vi "TagWrite.vi"(7 "LabVIEW Web Service Request":refnum<class "Web Request.lvclass">, 9 "value":T3="0", 10 "tagName":T1, 11 "type":T2) -> ()   [LabVIEW 2013]
uses:
  <vilib>/wsapi/Web Request.lvclass
  <vilib>/NI/TagWebClient/API/String Controls/value.ctl
  <vilib>/NI/TagWebClient/API/String Controls/type.ctl
  <vilib>/NI/TagWebClient/API/String Controls/tagName.ctl
  <vilib>/NI/Tag Bus/tag/Data Type.ctl
  <vilib>/NI/Tag Bus/table/data polymorphs/write one/write Double.vi
  <vilib>/NI/Tag Bus/table/data polymorphs/write one/write Single.vi
  <vilib>/NI/Tag Bus/table/data polymorphs/write one/write I64.vi
  <vilib>/NI/Tag Bus/table/data polymorphs/write one/write I32.vi
  <vilib>/NI/Tag Bus/table/data polymorphs/write one/write I16.vi
  <vilib>/NI/Tag Bus/table/data polymorphs/write one/write I8.vi
  <vilib>/NI/Tag Bus/table/data polymorphs/write one/write U64.vi
  <vilib>/NI/Tag Bus/table/data polymorphs/write one/write U32.vi
  <vilib>/NI/Tag Bus/table/data polymorphs/write one/write U16.vi
  <vilib>/NI/Tag Bus/table/data polymorphs/write one/write U8.vi
  <vilib>/NI/Tag Bus/table/data polymorphs/write one/write String.vi
  <vilib>/NI/Tag Bus/table/data polymorphs/write one/write Boolean.vi
  <vilib>/NI/Tag Bus/table/data table.lvlib
  <vilib>/NI/Tag Bus/tag/tag descriptor.lvclass
  <vilib>/NI/Tag Bus/dictionary/data dictionary.lvclass
  <vilib>/NI/TagWebClient/API/tagweb client API.lvlib
panel:
  # "Use the Web Service Request input terminal to call the VIs on the Web Services palette. Do not remove it from the connector pane unless you don't need access to the palette."
  # "Each additional control wired to the connector pane will be available as an input in the URL. To include an indicator in terminal-mode output (the default setting), it must also be wired to the connector pane."
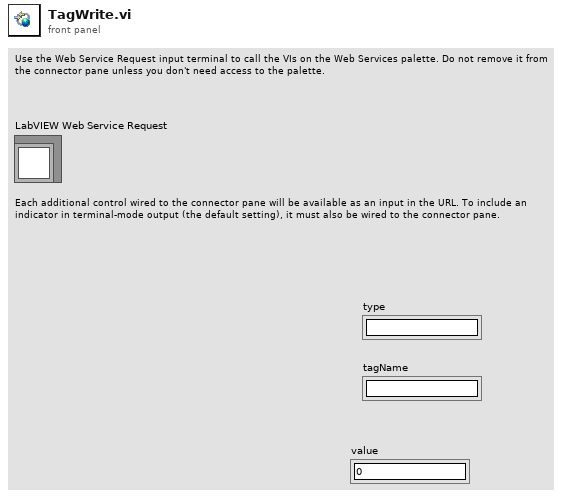
[diagram p1: front panel]
types:
  T1 = typedef "tagweb client API.lvlib/tagName.ctl" = string
  T2 = typedef "tagweb client API.lvlib/type.ctl" = string
  T3 = typedef "tagweb client API.lvlib/value.ctl" = string
  T4 = typedef "tag bus.lvlib/tag descriptor.lvclass/Data Type.ctl" = enum16{"Double", "Single", "I64", "I32", "I16", "I8", "U64", "U32", "U16", "U8", "Boolean", "String", "Array of Double", "Array of Single", "Array of I64", "Array of I32", "Array of I16", "Array of I8", "Array of U64", "Array of U32", "Array of U16", "Array of U8", "Array of Boolean", "Array of String"}
  T5 = typedef "tag bus.lvlib/data table.lvlib/data table.ctl" = cluster{"Double":dbl[], "Single":sgl[], "I64":i64[], "I32":i32[], "I16":i16[], "I8":i8[], "U64":u64[], "U32":u32[], "U16":u16[], "U8":u8[], "Boolean":bool[], "String":string[], "Array of Double":cluster{"DBL Array":dbl[]}[], "Array of Single":cluster{"SGL Array":sgl[]}[], "Array of I64":cluster{"I64 Array":i64[]}[], "Array of I32":cluster{"I32 Array":i32[]}[], "Array of I16":cluster{"I16 Array":i16[]}[], "Array of I8":cluster{"I8 Array":i8[]}[], "Array of U64":cluster{"U64 Array":u64[]}[], "Array of U32":cluster{"U32 Array":u32[]}[], "Array of U16":cluster{"U16 Array":u16[]}[], "Array of U8":cluster{"U8 Array":u8[]}[], "Array of Boolean":cluster{"Boolean Array":bool[]}[], "Array of String":cluster{"String Array":string[]}[]}
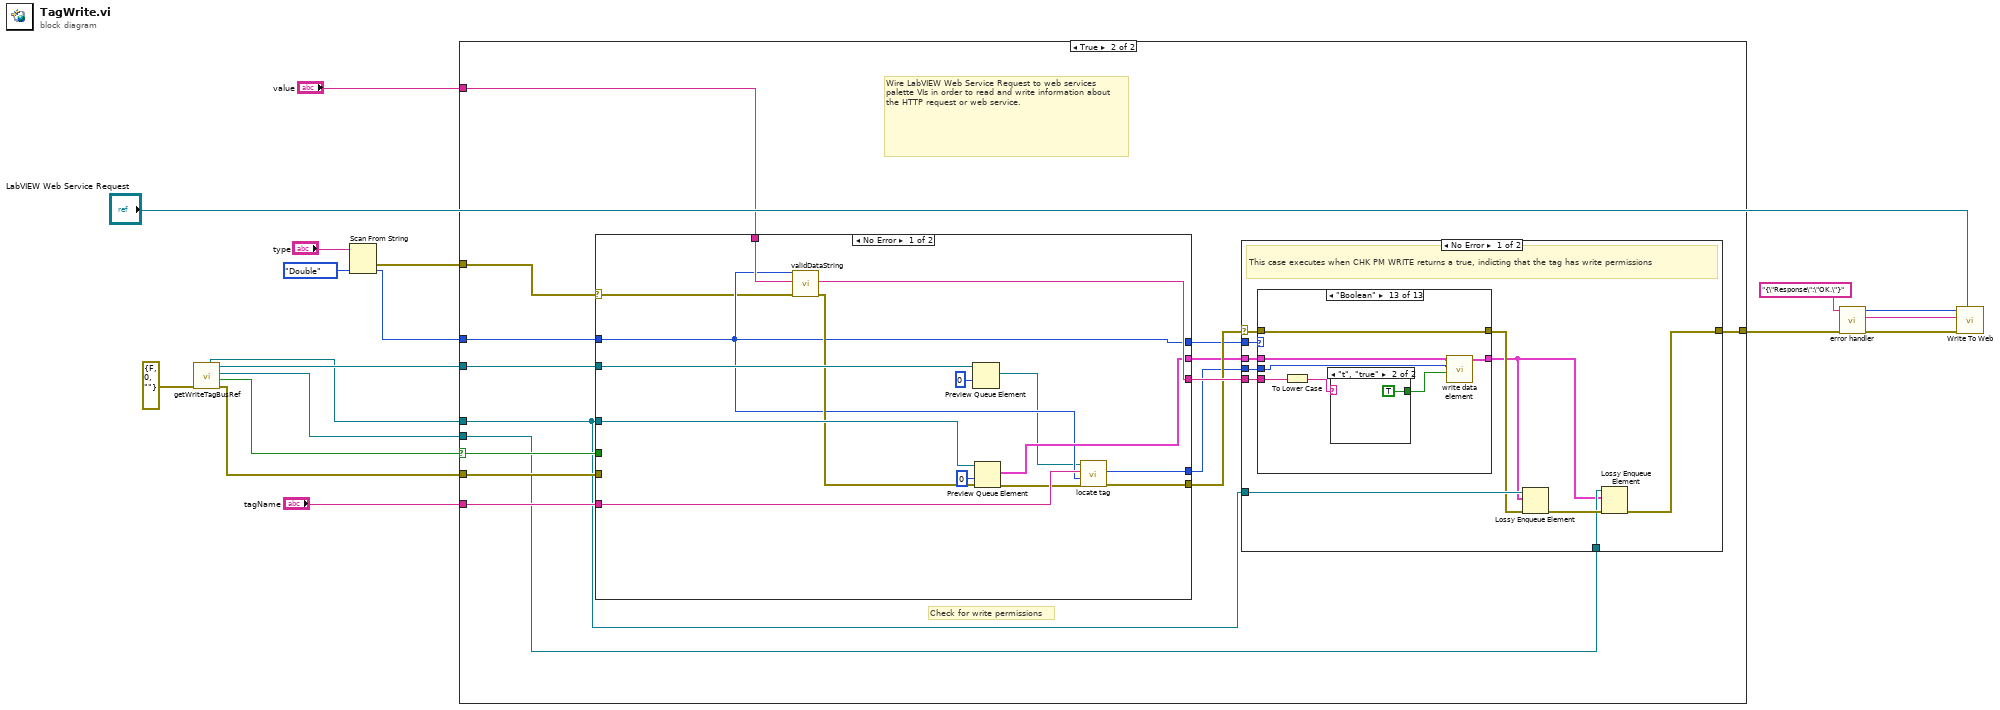
[diagram p0: block diagram]
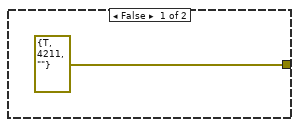
[diagram p2: hidden frame]
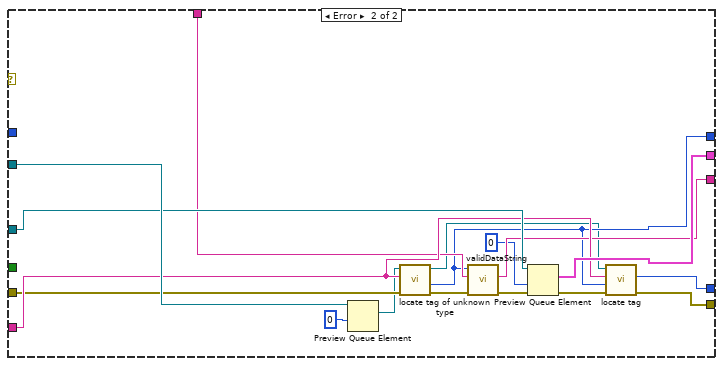
[diagram p3: hidden frame]
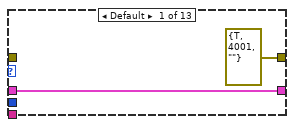
[diagram p4: hidden frame]
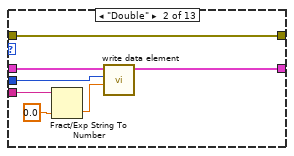
[diagram p5: hidden frame]
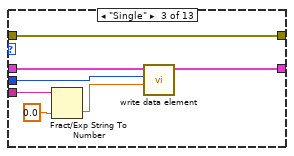
[diagram p6: hidden frame]
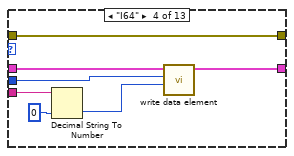
[diagram p7: hidden frame]
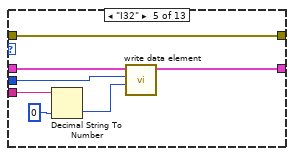
[diagram p8: hidden frame]
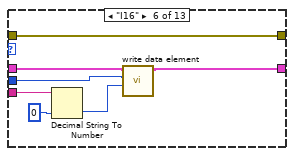
[diagram p9: hidden frame]
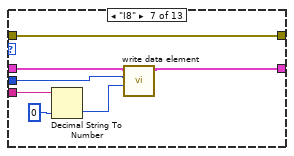
[diagram p10: hidden frame]
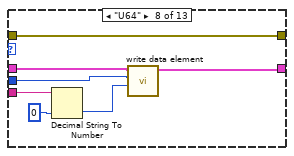
[diagram p11: hidden frame]
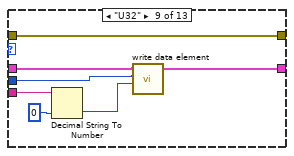
[diagram p12: hidden frame]
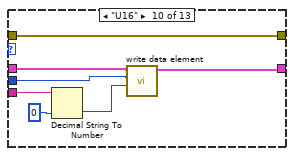
[diagram p13: hidden frame]
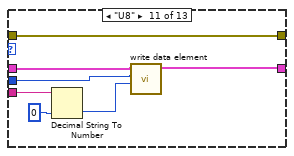
[diagram p14: hidden frame]
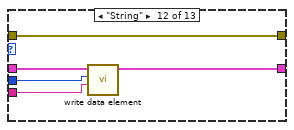
[diagram p15: hidden frame]
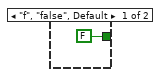
[diagram p16: hidden frame]
diagram:
  n1 = call "getWriteTagBusRef.vi"("error in"=errorcluster {"status"=FALSE, "code"=0, "source"=""} ("error in (no error)")) -> ("error out"=w14:errorcluster, "valid references"=w1:bool, "write tx data table"=w6:refnum<queue>, "write data dictionary"=w15:refnum<queue>, "actual write data table"=w7:refnum<queue>)  [unwired: 6 in]
  n2 = Scan From String(input string="type", default 1=Data_Type."Double" ("data type")) -> (error out=w9:errorcluster, output 1=w8:T4)  [unwired: 3 in, 2 out]
  n3 = case shown="True" w1 {
    selector: w1 -> [_ w22]
    tunnel: [errorcluster {"status"=TRUE, "code"=4211, "source"=""} ("error IO") w34] -> w18
    tunnel: w15 -> [_ w33]
    tunnel: w14 -> [_ w27]
    tunnel: "value" -> [_ w26]
    tunnel: "tagName" -> [_ w25]
    tunnel: w9 -> [_ w24]
    tunnel: w8 -> [_ w23]
    tunnel: w7 -> [_ w20]
    tunnel: w6 -> [_ w21]
    frame False {
    }
    frame True {
      # "Check for write permissions"
      # "Wire LabVIEW Web Service Request to web services palette VIs in order to read and write information about the HTTP request or web service."
      n4 = case shown="No Error" w24 {
        selector: w24 -> [w35 _]
        tunnel: w26 -> [w49 w60]
        tunnel: w33 -> [w48 w66]
        tunnel: w20 -> [w47 w65]
        tunnel: [w46 w59] -> w32
        tunnel: w22 -> [_ _]
        tunnel: w25 -> [w44 w61]
        tunnel: [w43 w64] -> w31
        tunnel: [w40 w58] -> w30
        tunnel: [w42 w63] -> w29
        tunnel: [w41 w62] -> w28
        tunnel: w27 -> [_ w57]
        tunnel: w23 -> [w40 _]
        frame No Error {
          n5 = call "validDataString.vi"("error in (no error)"=w35, "value in"=w49, "data type"=w40) -> ("error out"=w45:errorcluster, "value out"=w46:string)  [unwired: 6 in, 1 out]
          n6 = Preview Queue Element(queue=w48, timeout in ms (-1)=0) -> (element=w36:refnum<class "data dictionary.lvclass">)  [unwired: 1 in, 3 out]
          n7 = Preview Queue Element(queue=w47, timeout in ms (-1)=0, error in (no error)=w45) -> (element=w41:T5, error out=w38:errorcluster)  [unwired: 2 out]
          n8 = call <vilib>:"locate tag.vi"("error in"=w38, "data type"=w40, "name"=w44, "data dictionary in"=w36) -> ("error out"=w43:errorcluster, "index"=w42:i32)  [unwired: 5 in, 1 out]
        }
        frame Error {
          n9 = Preview Queue Element(queue=w66, timeout in ms (-1)=0) -> (element=w50:refnum<class "data dictionary.lvclass">)  [unwired: 1 in, 3 out]
          n10 = call <vilib>:"locate tag of unknown type.vi"("error in"=w57, "name"=w61, "data dictionary in"=w50) -> ("error out"=w52:errorcluster, "data type"=w58:T4, "data dictionary out"=w51:refnum<class "data dictionary.lvclass">)  [unwired: 5 in, 1 out]
          n11 = call "validDataString.vi"("error in (no error)"=w52, "value in"=w60, "data type"=w58) -> ("error out"=w53:errorcluster, "value out"=w59:string)  [unwired: 6 in, 1 out]
          n12 = Preview Queue Element(queue=w65, timeout in ms (-1)=0, error in (no error)=w53) -> (element=w62:T5, error out=w55:errorcluster)  [unwired: 2 out]
          n13 = call <vilib>:"locate tag.vi"("error in"=w55, "data type"=w58, "name"=w61, "data dictionary in"=w51) -> ("error out"=w64:errorcluster, "index"=w63:i32)  [unwired: 5 in, 1 out]
        }
      }
      n14 = case shown="No Error" w31 {
        selector: w31 -> [w73 w164]
        tunnel: w32 -> [w77 _]
        tunnel: w29 -> [w76 _]
        tunnel: [w69 w164] -> w34
        tunnel: w30 -> [w75 _]
        tunnel: w28 -> [w74 _]
        tunnel: w20 -> [w72 _]
        tunnel: w21 -> [w68 _]
        frame No Error {
          # "This case executes when CHK PM WRITE returns a true, indicting that the tag has write permissions"
          n15 = case shown="\"Boolean\"" w75 {
            tunnel: w76 -> [_ w83 w88 w95 w102 w109 w116 w124 w131 w137 w144 w152 w156]
            tunnel: [errorcluster {"status"=TRUE, "code"=4001, "source"=""} ("error out") w81 w91 w98 w105 w112 w119 w126 w133 w140 w147 w154 w159] -> w71
            tunnel: w77 -> [_ w86 w93 w100 w107 w114 w121 w128 w135 w142 w149 w151 w161]
            tunnel: w74 -> [w78 w84 w90 w97 w103 w110 w117 w125 w132 w139 w145 w153 w158]
            tunnel: w73 -> [_ w81 w91 w98 w105 w112 w119 w126 w133 w140 w147 w154 w159]
            tunnel: [w78 w80 w89 w96 w104 w111 w118 w122 w129 w138 w146 w150 w157] -> w67
            frame Default {
            }
            frame "Double" {
              n16 = Fract/Exp String To Number(string=w86, default (0 dbl)=0.0 ("Value")) -> (number=w82:dbl)  [unwired: 2 in, 1 out]
              n17 = call-poly <vilib>:"write data element.vi"("value"=w82, "index"=w83, "data table in"=w84) -> ("data table out"=w80:T5)  [unwired: 8 in]
            }
            frame "Single" {
              n18 = Fract/Exp String To Number(string=w93, default (0 dbl)=sgl 0.0 ("Value")) -> (number=w87:sgl)  [unwired: 2 in, 1 out]
              n19 = call-poly <vilib>:"write data element.vi"("value"=w87, "index"=w88, "data table in"=w90) -> ("data table out"=w89:T5)  [unwired: 8 in]
            }
            frame "I64" {
              n20 = Decimal String To Number(string=w100, default (0L)=i64 0 ("Value")) -> (number=w94:i64)  [unwired: 1 in, 1 out]
              n21 = call-poly <vilib>:"write data element.vi"("value"=w94, "index"=w95, "data table in"=w97) -> ("data table out"=w96:T5)  [unwired: 8 in]
            }
            frame "I32" {
              n22 = Decimal String To Number(string=w107, default (0L)=0 ("Value")) -> (number=w101:i32)  [unwired: 1 in, 1 out]
              n23 = call-poly <vilib>:"write data element.vi"("value"=w101, "index"=w102, "data table in"=w103) -> ("data table out"=w104:T5)  [unwired: 8 in]
            }
            frame "I16" {
              n24 = Decimal String To Number(string=w114, default (0L)=i16 0 ("Value")) -> (number=w108:i16)  [unwired: 1 in, 1 out]
              n25 = call-poly <vilib>:"write data element.vi"("value"=w108, "index"=w109, "data table in"=w110) -> ("data table out"=w111:T5)  [unwired: 8 in]
            }
            frame "I8" {
              n26 = Decimal String To Number(string=w121, default (0L)=i8 0 ("Value")) -> (number=w115:i8)  [unwired: 1 in, 1 out]
              n27 = call-poly <vilib>:"write data element.vi"("value"=w115, "index"=w116, "data table in"=w117) -> ("data table out"=w118:T5)  [unwired: 8 in]
            }
            frame "U64" {
              n28 = Decimal String To Number(string=w128, default (0L)=u64 0 ("Value")) -> (number=w123:u64)  [unwired: 1 in, 1 out]
              n29 = call-poly <vilib>:"write data element.vi"("value"=w123, "index"=w124, "data table in"=w125) -> ("data table out"=w122:T5)  [unwired: 8 in]
            }
            frame "U32" {
              n30 = Decimal String To Number(string=w135, default (0L)=u32 0 ("Value")) -> (number=w130:u32)  [unwired: 1 in, 1 out]
              n31 = call-poly <vilib>:"write data element.vi"("value"=w130, "index"=w131, "data table in"=w132) -> ("data table out"=w129:T5)  [unwired: 8 in]
            }
            frame "U16" {
              n32 = Decimal String To Number(string=w142, default (0L)=u16 0 ("Value")) -> (number=w136:u16)  [unwired: 1 in, 1 out]
              n33 = call-poly <vilib>:"write data element.vi"("value"=w136, "index"=w137, "data table in"=w139) -> ("data table out"=w138:T5)  [unwired: 8 in]
            }
            frame "U8" {
              n34 = Decimal String To Number(string=w149, default (0L)=u8 0 ("Value")) -> (number=w143:u8)  [unwired: 1 in, 1 out]
              n35 = call-poly <vilib>:"write data element.vi"("value"=w143, "index"=w144, "data table in"=w145) -> ("data table out"=w146:T5)  [unwired: 8 in]
            }
            frame "String" {
              n36 = call-poly <vilib>:"write data element.vi"("value"=w151, "index"=w152, "data table in"=w153) -> ("data table out"=w150:T5)  [unwired: 8 in]
            }
            frame "Boolean" {
              n37 = To Lower Case(string=w161) -> (all lower case string=w160:string)
              n38 = case shown="\"t\", \"true\"" w160 {
                tunnel: [FALSE ("Value") TRUE ("Value")] -> w155
                frame "f", "false", Default {
                }
                frame "t", "true" {
                }
              }
              n39 = call-poly <vilib>:"write data element.vi"("value"=w155, "index"=w156, "data table in"=w158) -> ("data table out"=w157:T5)  [unwired: 8 in]
            }
          }
          n40 = Lossy Enqueue Element(queue=w72, element=w67, error in (no error)=w71) -> (error out=w70:errorcluster)  [unwired: 3 out]
          n41 = Lossy Enqueue Element(queue=w68, element=w67, error in (no error)=w70) -> (error out=w69:errorcluster)  [unwired: 3 out]
        }
        frame Error {
          # "This case executes when CHK PM WRITE returns a false, indicating that the tag does not have write permissions"
        }
      }
    }
  }
  n42 = call "error handler.vi"("error in (no error)"=w18, "Success Message"="{\"Response\":\"OK.\"}" ("response string")) -> ("error out"=w4:errorcluster, "Response String"=w2:string, "Response Code"=w3:i32)  [unwired: 7 in]
  n43 = call <vilib>:"Write To Web.vi"("Web Request in"="LabVIEW Web Service Request", "error in (no error)"=w4, "Response String"=w2, "Response Code"=w3) -> ()  [unwired: 7 in, 1 out]
